vi "Set Items.vi"(8 "error in (no error)":errorcluster caption="错误输入（无错误）", 10 "Items":refnum<data-value>[](array[refnum]), 11 "Section输入":refnum<class "Section.lvclass">) -> (0 "error out":errorcluster caption="错误输出", 3 "Section输出":refnum<class "Section.lvclass">)   [LabVIEW 2013, in "Hierarchy Framework.lvlib" / "Section.lvclass"]
uses:
  Section.lvclass
  Item/Item.lvclass
  Section.lvclass/Section.ctl
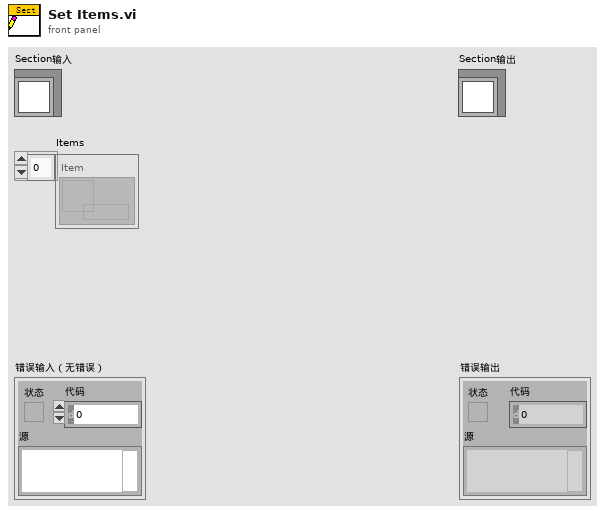
[diagram p1: front panel]
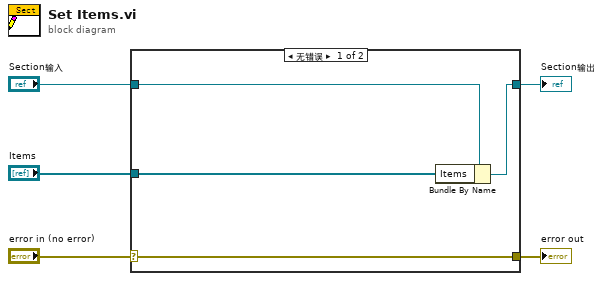
[diagram p0: block diagram]
diagram:
  n1 = case shown="无错误" "error in (no error)" {
    selector: "error in (no error)" -> [w9 w10]
    tunnel: [w9 w10] -> w4
    tunnel: [w8 w11] -> w2
    tunnel: "Section输入" -> [w6 w11]
    tunnel: "Items" -> [w7 _]
    frame No Error {
      n2 = Bundle By Name(cluster=w6, "Items"=w7) -> (w8:refnum<class "Section.lvclass">)
    }
    frame Error {
    }
  }
  "error out" <- w4
  "Section输出" <- w2
